vi "number_to_b36.vi"(1 "Number":i32) -> (0 "Base36 string":string)   [LabVIEW 2023]
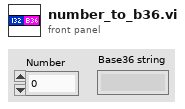
[diagram p1: front panel]
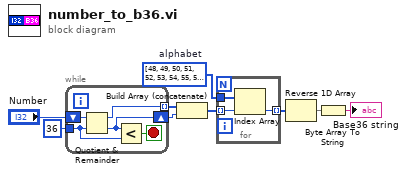
[diagram p0: block diagram]
diagram:
  w3 = u8[] [48, 49, 50, 51, 52, 53, 54, 55, 56, 57, 97, 98, 99, 100, 101, 102, 103, 104, 105, 106, 107, 108, 109, 110, 111, 112, 113, 114, 115, 116, 117, 118, 119, 120, 121, 122]  # alphabet
  n1 = while {
    shift-right: [w12] -> w8
    shift-left: "Number" -> [w14]
    tunnel: 36 ("y") -> [w13]
    tunnel: [w11] -> w9 mode=indexing
    stop <- w10 stop-if-true
    n2 = Quotient & Remainder(x=w14, y=w13) -> (x-y*floor(x/y)=w11:i32, floor(x/y)=w12:i32)
    n3 = Less?(x=w12, y=w13) -> (x < y?=w10:bool)
  }
  n4 = Build Array (concatenate)(w9, w8) -> (w7:i32[])
  n5 = for {
    tunnel: w3 -> [w17]
    tunnel: w7 -> [w16] mode=indexing
    tunnel: [w15] -> w6 mode=indexing
    n6 = Index Array(array=w17, index=w16) -> (element=w15:u8)
  }
  n7 = Reverse 1D Array(array=w6) -> (reversed array=w5:u8[])
  n8 = Byte Array To String(unsigned byte array=w5) -> (string=→"Base36 string":string)
